vi "S2C_FPGA_Main.vi"() -> ()   [LabVIEW 2015]
uses:
  <vilib>/rvi/Emulation/niFpgaGetClockAttributes.vi
  <vilib>/rvi/Emulation/niFpgaSctlEmulationGetInTimedLoop.vi
  <vilib>/rvi/Emulation/niFpgaEmulationReportErrorSimple.vi
  <vilib>/rvi/Emulation/niFpgaCriticalErrorInLSC.vi
  <vilib>/rvi/eio/common/nirviEmuTemplateMethod_errors.vi
  S2C_FPGA_Global.vi
  <vilib>/eio/EIONode/EIONode.xnode
panel:
  out "Conn0/AI7":i16 min=-10 max=10 format="%04x"
  out "Conn0/AI6":i16 min=-10 max=10 format="%04x"
  out "Conn0/AI5":i16 min=-10 max=10 format="%04x"
  out "Conn0/AI4":i16 min=-10 max=10 format="%04x"
  out "Conn0/AI3":i16 min=-10 max=10 format="%04x"
  out "Conn0/AI2":i16 min=-10 max=10 format="%04x"
  out "Conn0/AI1":i16 min=-10 max=10 format="%04x"
  out "Conn0/AI0":i16 min=-10 max=10 format="%04x"
  in  "Conn0/AO7":i16 format="%04x"
  in  "Conn0/AO6":i16 format="%04x"
  in  "Conn0/AO5":i16 format="%04x"
  in  "Conn0/AO4":i16 format="%04x"
  in  "Conn0/AO3":i16 format="%04x"
  in  "Conn0/AO2":i16 format="%04x"
  in  "Conn0/AO1":i16 format="%04x"
  in  "Conn0/AO0":i16 format="%04x"
  out "Conn0/Port1":u8 format="%08b"
  out "Conn0/Port0":u8 format="%08b"
  out "Conn2/Port4":u8 format="%08b"
  out "Conn2/Port3":u8 format="%08b"
  out "Conn2/Port2":u8 format="%08b"
  out "Conn2/Port1":u8 format="%08b"
  out "Conn2/Port0":u8 format="%08b"
  out "Conn1/Port4":u8 format="%08b"
  out "Conn1/Port3":u8 format="%08b"
  out "Conn1/Port2":u8 format="%08b"
  out "Conn1/Port1":u8 format="%08b"
  out "Conn1/Port0":u8 format="%08b"
  # "Digital Input/Output"
  # "Analog Input/Output"
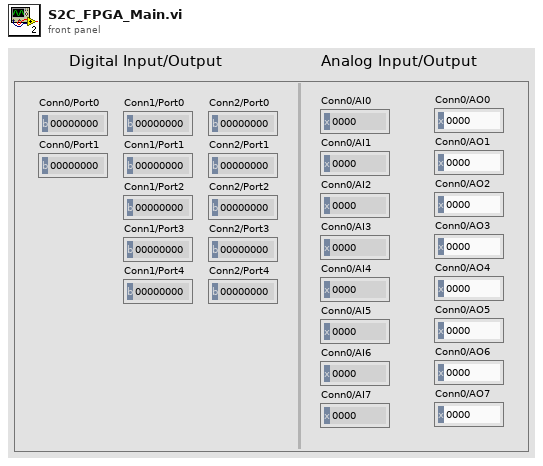
[diagram p1: front panel]
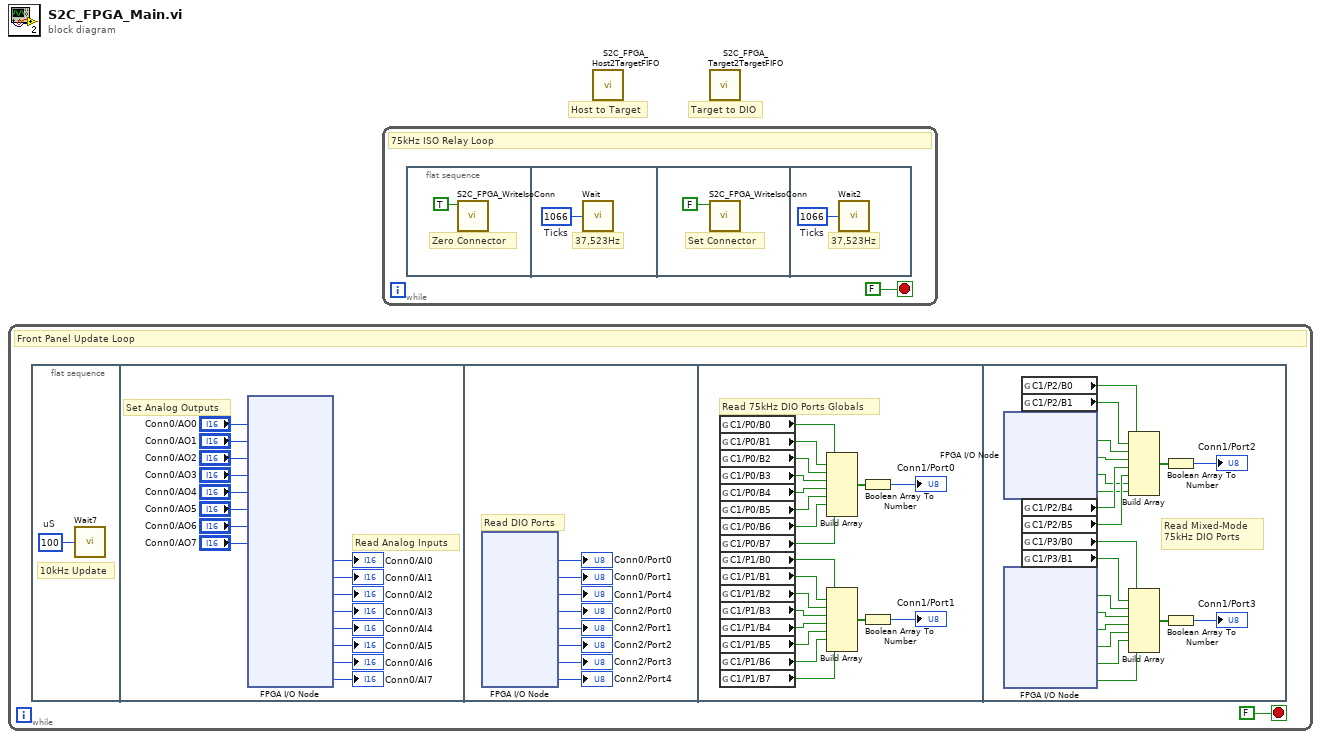
[diagram p0: block diagram]
diagram:
  # "Target to DIO"
  # "Host to Target"
  n1 = while {
    stop <- FALSE stop-if-true
    # "Front Panel Update Loop"
    n2 = flat-sequence {
      frame #0 {
        w2 = u8 100  # uS
        # "10kHz Update"
        n3 = call "Wait7"("Count(uSec)"=w2) -> ()  [unwired: 1 out]
      }
      frame #1 {
        # "Read Analog Inputs"
        # "Set Analog Outputs"
        n4 = xnode "FPGA I/O Node"("C0/AO0"="Conn0/AO0", "C0/AO1"="Conn0/AO1", "C0/AO2"="Conn0/AO2", "C0/AO3"="Conn0/AO3", "C0/AO4"="Conn0/AO4", "C0/AO5"="Conn0/AO5", "C0/AO6"="Conn0/AO6", "C0/AO7"="Conn0/AO7") -> ("C0/AI0"=→"Conn0/AI0":i16, "C0/AI1"=→"Conn0/AI1":i16, "C0/AI2"=→"Conn0/AI2":i16, "C0/AI3"=→"Conn0/AI3":i16, "C0/AI4"=→"Conn0/AI4":i16, "C0/AI5"=→"Conn0/AI5":i16, "C0/AI6"=→"Conn0/AI6":i16, "C0/AI7"=→"Conn0/AI7":i16)  [unwired: 16 in, 16 out]
      }
      frame #2 {
        # "Read DIO Ports"
        n5 = xnode "FPGA I/O Node"() -> ("C0/P0"=→"Conn0/Port0":u8, "C0/P1"=→"Conn0/Port1":u8, "C1/P4"=→"Conn1/Port4":u8, "C2/P0"=→"Conn2/Port0":u8, "C2/P1"=→"Conn2/Port1":u8, "C2/P2"=→"Conn2/Port2":u8, "C2/P3"=→"Conn2/Port3":u8, "C2/P4"=→"Conn2/Port4":u8)  [unwired: 8 in, 8 out]
      }
      frame #3 {
        # "Read 75kHz DIO Ports Globals"
        n6 = global read "S2C_FPGA_Global.vi" "C1/P0/B0"() -> (w29:bool)
        n7 = global read "S2C_FPGA_Global.vi" "C1/P0/B1"() -> (w30:bool)
        n8 = global read "S2C_FPGA_Global.vi" "C1/P0/B2"() -> (w31:bool)
        n9 = global read "S2C_FPGA_Global.vi" "C1/P0/B3"() -> (w32:bool)
        n10 = global read "S2C_FPGA_Global.vi" "C1/P0/B4"() -> (w33:bool)
        n11 = global read "S2C_FPGA_Global.vi" "C1/P0/B5"() -> (w34:bool)
        n12 = global read "S2C_FPGA_Global.vi" "C1/P0/B6"() -> (w35:bool)
        n13 = global read "S2C_FPGA_Global.vi" "C1/P0/B7"() -> (w36:bool)
        n14 = global read "S2C_FPGA_Global.vi" "C1/P1/B0"() -> (w46:bool)
        n15 = global read "S2C_FPGA_Global.vi" "C1/P1/B1"() -> (w45:bool)
        n16 = global read "S2C_FPGA_Global.vi" "C1/P1/B2"() -> (w44:bool)
        n17 = global read "S2C_FPGA_Global.vi" "C1/P1/B3"() -> (w43:bool)
        n18 = global read "S2C_FPGA_Global.vi" "C1/P1/B4"() -> (w42:bool)
        n19 = global read "S2C_FPGA_Global.vi" "C1/P1/B5"() -> (w41:bool)
        n20 = global read "S2C_FPGA_Global.vi" "C1/P1/B6"() -> (w40:bool)
        n21 = global read "S2C_FPGA_Global.vi" "C1/P1/B7"() -> (w39:bool)
        n22 = Build Array(w29, w30, w31, w32, w33, w34, w35, w36) -> (w37:bool[])
        n23 = Build Array(w46, w45, w44, w43, w42, w41, w40, w39) -> (w38:bool[])
        n24 = Boolean Array To Number(Boolean array=w37) -> (number=→"Conn1/Port0":u8)
        n25 = Boolean Array To Number(Boolean array=w38) -> (number=→"Conn1/Port1":u8)
      }
      frame #4 {
        # "Read Mixed-Mode\n75kHz DIO Ports"
        n26 = xnode "FPGA I/O Node"() -> ("C1/P2/B2"=w55:bool, "C1/P2/B3"=w56:bool, "C1/P2/B6"=w48:bool, "C1/P2/B7"=w47:bool)  [unwired: 4 in, 4 out]
        n27 = xnode "FPGA I/O Node"() -> ("C1/P3/B2"=w60:bool, "C1/P3/B3"=w61:bool, "C1/P3/B4"=w62:bool, "C1/P3/B5"=w63:bool, "C1/P3/B6"=w64:bool, "C1/P3/B7"=w65:bool)  [unwired: 6 in, 6 out]
        n28 = global read "S2C_FPGA_Global.vi" "C1/P2/B0"() -> (w53:bool)
        n29 = global read "S2C_FPGA_Global.vi" "C1/P2/B1"() -> (w54:bool)
        n30 = global read "S2C_FPGA_Global.vi" "C1/P2/B4"() -> (w50:bool)
        n31 = global read "S2C_FPGA_Global.vi" "C1/P2/B5"() -> (w49:bool)
        n32 = global read "S2C_FPGA_Global.vi" "C1/P3/B0"() -> (w58:bool)
        n33 = global read "S2C_FPGA_Global.vi" "C1/P3/B1"() -> (w59:bool)
        n34 = Build Array(w53, w54, w55, w56, w50, w49, w48, w47) -> (w57:bool[])
        n35 = Build Array(w58, w59, w60, w61, w62, w63, w64, w65) -> (w66:bool[])
        n36 = Boolean Array To Number(Boolean array=w57) -> (number=→"Conn1/Port2":u8)
        n37 = Boolean Array To Number(Boolean array=w66) -> (number=→"Conn1/Port3":u8)
      }
    }
  }
  n38 = while {
    stop <- FALSE stop-if-true
    # "75kHz ISO Relay Loop"
    n39 = flat-sequence {
      frame #0 {
        # "Zero Connector"
        n40 = call "S2C_FPGA_WriteIsoConn.vi"("Reset"=TRUE) -> ()  [unwired: 11 in]
      }
      frame #1 {
        w69 = u16 1066  # Ticks
        # "37,523Hz"
        n41 = call "Wait"("Count(Ticks)"=w69) -> ()  [unwired: 1 out]
      }
      frame #2 {
        # "Set Connector"
        n42 = call "S2C_FPGA_WriteIsoConn.vi"("Reset"=FALSE) -> ()  [unwired: 11 in]
      }
      frame #3 {
        w71 = u16 1066  # Ticks
        # "37,523Hz"
        n43 = call "Wait2"("Count(Ticks)"=w71) -> ()  [unwired: 1 out]
      }
    }
  }
  n44 = call "S2C_FPGA_Host2TargetFIFO.vi"() -> ()  [unwired: 12 in]
  n45 = call "S2C_FPGA_Target2TargetFIFO.vi"() -> ()  [unwired: 12 in]
